vi "redo.vi"(8 "error in (no error)":errorcluster, 11 "ScriptEditorV2 in":refnum<class "ScriptEditorV2.lvclass">) -> (0 "error out":errorcluster, 3 "ScriptEditorV2 out":refnum<class "ScriptEditorV2.lvclass">)   [LabVIEW 2011, in "Views.lvlib" / "ScriptEditor.lvlib" / "ScriptEditorV2.lvclass"]
uses:
  ScriptEditorV2.lvclass
  ScriptEditorV2.lvclass/ScriptEditorV2.ctl
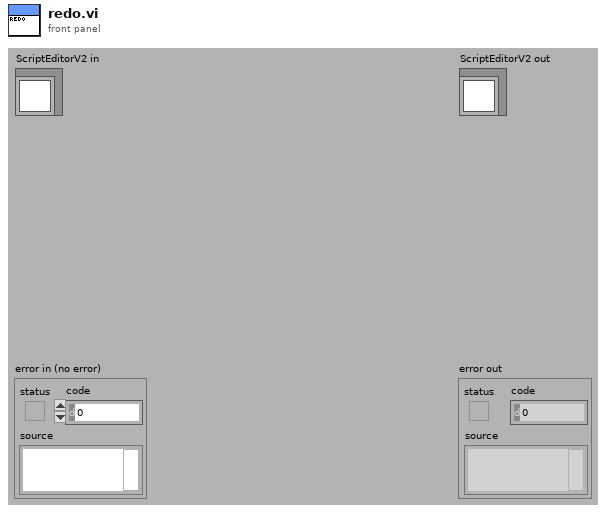
[diagram p1: front panel]
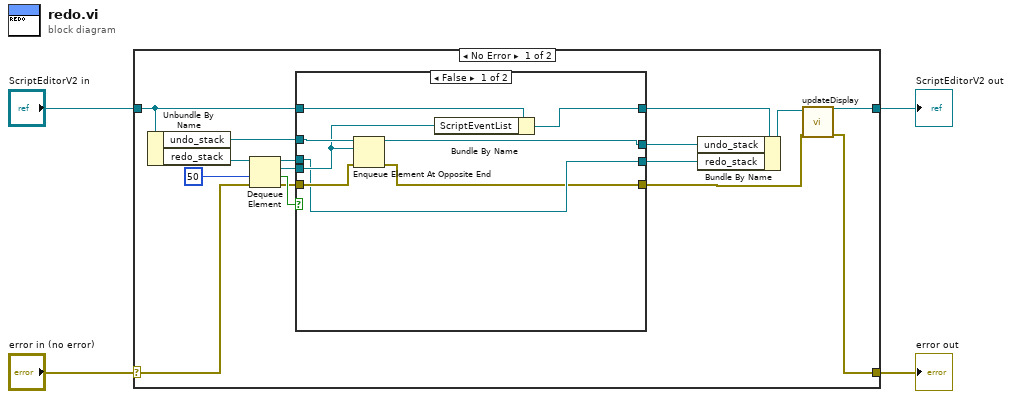
[diagram p0: block diagram]
diagram:
  n1 = case shown="No Error" "error in (no error)" {
    selector: "error in (no error)" -> [w10 w34]
    tunnel: [w5 w34] -> w3
    tunnel: [w8 w33] -> w1
    tunnel: "ScriptEditorV2 in" -> [w13 w33]
    frame No Error {
      n2 = Unbundle By Name(w13) -> ("undo_stack"=w16:refnum<queue>, "redo_stack"=w19:refnum<queue>)
      n3 = Dequeue Element(queue=w19, timeout in ms (-1)=50, error in (no error)=w10) -> (queue out=w18:refnum<queue>, element=w15:refnum<class "ScriptEventList.lvclass">, timed out?=w20:bool, error out=w14:errorcluster)
      n4 = case shown="False" w20 {
        tunnel: w18 -> [w23 w30]
        tunnel: w16 -> [w28 w31]
        tunnel: w15 -> [w25 _]
        tunnel: w14 -> [w27 w29]
        tunnel: w13 -> [w26 w32]
        tunnel: [w24 w32] -> w9
        tunnel: [w22 w31] -> w12
        tunnel: [w23 w30] -> w11
        tunnel: [w21 w29] -> w6
        frame False {
          n5 = Enqueue Element At Opposite End(queue=w28, element=w25, error in (no error)=w27) -> (queue out=w22:refnum<queue>, error out=w21:errorcluster)  [unwired: 1 in, 1 out]
          n6 = Bundle By Name(cluster=w26, "ScriptEventList"=w25) -> (w24:refnum<class "ScriptEditorV2.lvclass">)
        }
        frame True {
        }
      }
      n7 = Bundle By Name(cluster=w9, "undo_stack"=w12, "redo_stack"=w11) -> (w7:refnum<class "ScriptEditorV2.lvclass">)
      n8 = call "updateDisplay.vi"("error in (no error)"=w6, "ScriptEditorV2 in"=w7) -> ("error out"=w5:errorcluster, "ScriptEditorV2 out"=w8:refnum<class "ScriptEditorV2.lvclass">)  [unwired: 8 in]
    }
    frame Error {
    }
  }
  "error out" <- w3
  "ScriptEditorV2 out" <- w1
